vi "tcs_putSample_kernelTrackRefSys.vi"(8 "error in (no error)":errorcluster, 11 "kernel_TrackRefSys_Ctl":T1={"ae2mt[9]"=[0.0, 0.0, 0.0, 0.0, 0.0, 0.0, 0.0, 0.0, 0.0], "amprms[21]"=[0.0, 0.0, 0.0, 0.0, 0.0, 0.0, 0.0, 0.0, 0.0, 0.0, 0.0, 0.0, 0.0, 0.0, 0.0, 0.0, 0.0, 0.0, 0.0, 0.0, 0.0], "cst"=0.0, "diurab"=0.0, "hm"=0.0, "humid"=0.0, "press"=0.0, "refa"=0.0, "refb"=0.0, "sst"=0.0, "tdbj"=0.0, "temp"=0.0, "tlat"=0.0, "tlr"=0.0, "wavel"=0.0}) -> (0 "error out":errorcluster, 2 "function return":i32, 3 "kernel_TrackRefSys_Ctl out":T1)   [LabVIEW 2016, in "SALLV_tcs.lvlib"]
doc: "int tcs_shm_putSample_kernel_TrackRefSysLV(tcs_kernel_TrackRefSysLV *kernel_TrackRefSys_Ctl );"
uses:
  SALLV_tcs.lvlib
  DataTypes/kernel_TrackRefSys.ctl
  SALLV_tcs.so
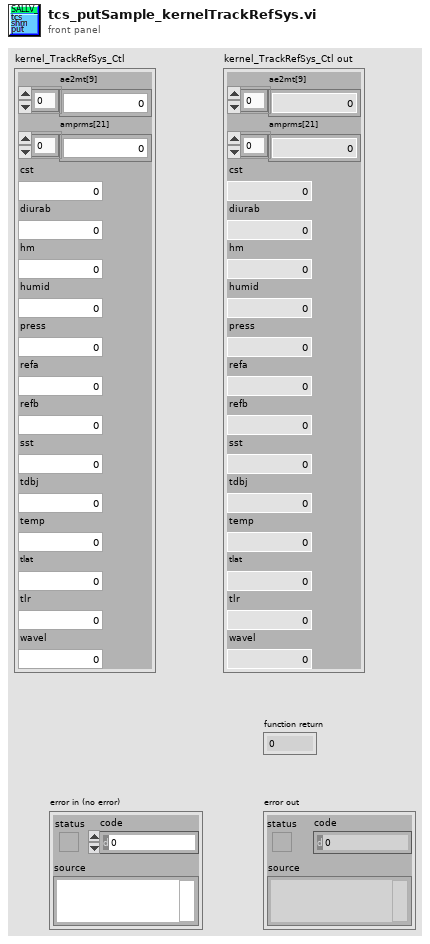
[diagram p1: front panel]
types:
  T1 = typedef "SALLV_tcs.lvlib/kernel_TrackRefSys.ctl" = cluster{"ae2mt[9]":sgl[], "amprms[21]":sgl[], "cst":sgl, "diurab":sgl, "hm":sgl, "humid":sgl, "press":sgl, "refa":sgl, "refb":sgl, "sst":sgl, "tdbj":sgl, "temp":sgl, "tlat":sgl, "tlr":sgl, "wavel":sgl}
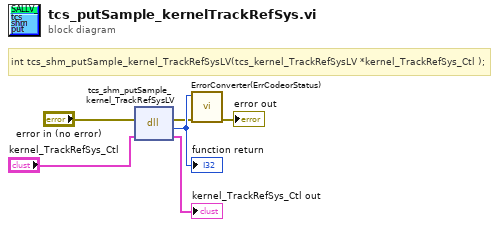
[diagram p0: block diagram]
diagram:
  # "int tcs_shm_putSample_kernel_TrackRefSysLV(tcs_kernel_TrackRefSysLV *kernel_TrackRefSys_Ctl );"
  n1 = dll-call lib="home/andres/Desktop/SALLV_tcs/SALLV_tcs.*" fn="tcs_shm_putSample_kernel_TrackRefSysLV"(error in="error in (no error)", "kernel_TrackRefSys_Ctl"="kernel_TrackRefSys_Ctl") -> (error out=w2:errorcluster, w6:i32, "kernel_TrackRefSys_Ctl"=→"kernel_TrackRefSys_Ctl out":T1)  [unwired: 2 in, 1 out]
  "function return" <- w6
  n2 = call "ErrorConverter(ErrCodeorStatus).vi"("error in (no error)"=w2, "error code"=w6) -> ("error out"=→"error out":errorcluster)  [unwired: 9 in]
